vi "SelRess.vi"(5 "Instr":bool=TRUE, 6 "UsedRess":string[](array[string]), 7 "RessName":string caption="RessourceName", 8 "ErrorIn(No Error)":errorcluster caption="entrée d'erreur (pas d'erreur)", 9 "InstrNames":string[](array[string]), 10 "RessArray":string[][](array[string]), 11 "InstrName":string caption="Instrument Name") -> (0 "sortie d'erreur":errorcluster, 1 "RessAlias":string, 2 "RessNameOut":string, 3 "InstrNameOut":string, 4 "Cancel Out":bool)   [LabVIEW 2019]
uses:
  SelRessState.ctl
  <vilib>/Utility/miscctls.llb/LVRectTypeDef.ctl
panel:
  out "InstStep":string
  in  "Cancel":bool
  in  "Add":bool
  in  "Ressources":i32(listbox)
  # "1. Choose a ressource from the list to communicate with the Instrument\nor enter a ressource name manually"
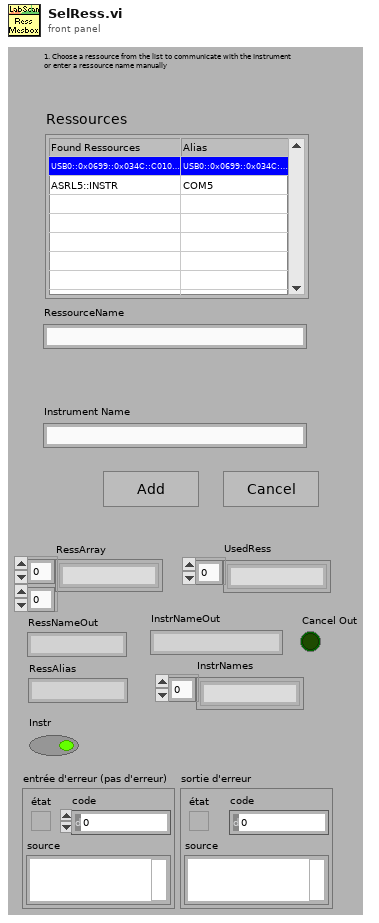
[diagram p1: front panel]
types:
  T1 = typedef "SelRessState.ctl" = enum16{"InitProg", "InstrNameExist?", "RessNameExist?", "RessInUse?", "RessSelected", "Cancel"}
  T2 = enum8{"Enabled", "Disabled", "Disabled and Grayed Out"}
  T3 = typedef "LVRectTypeDef.ctl" = cluster{"Left":i16, "Top":i16, "Right":i16, "Bottom":i16}
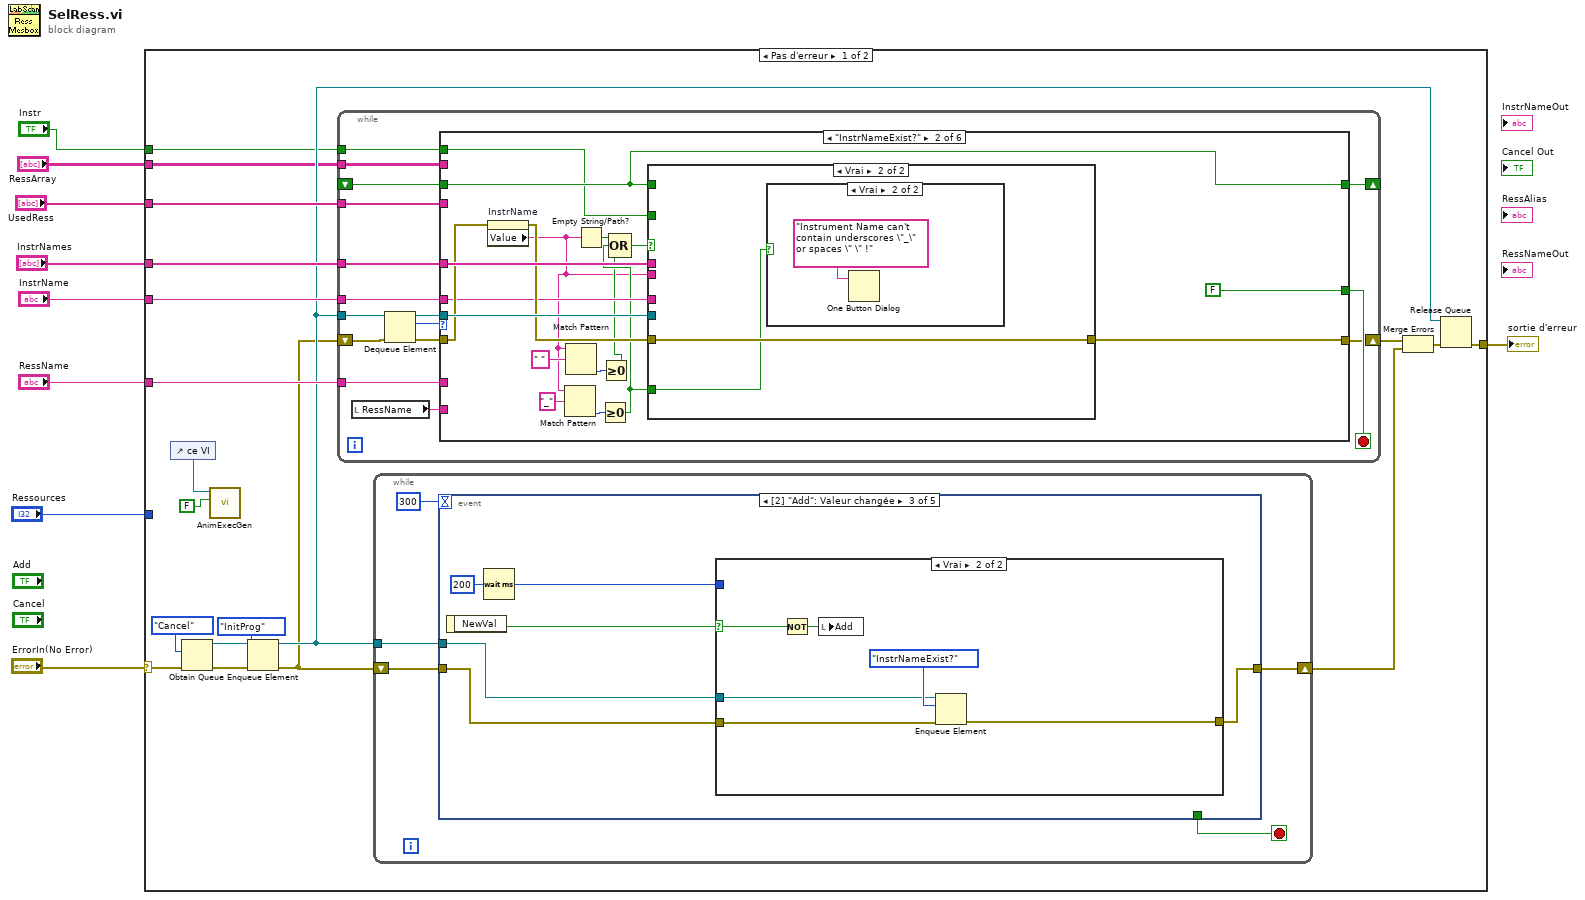
[diagram p0: block diagram]
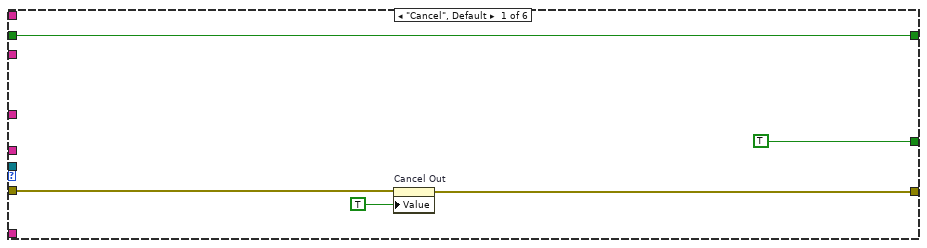
[diagram p2: hidden frame]
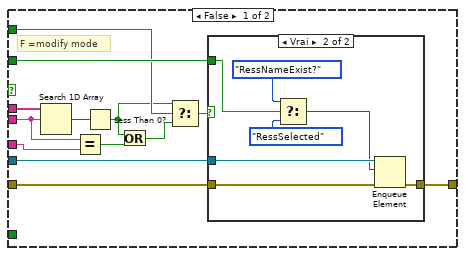
[diagram p3: hidden frame]
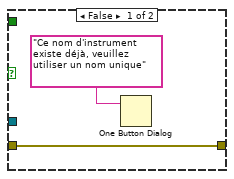
[diagram p4: hidden frame]
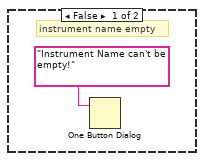
[diagram p5: hidden frame]
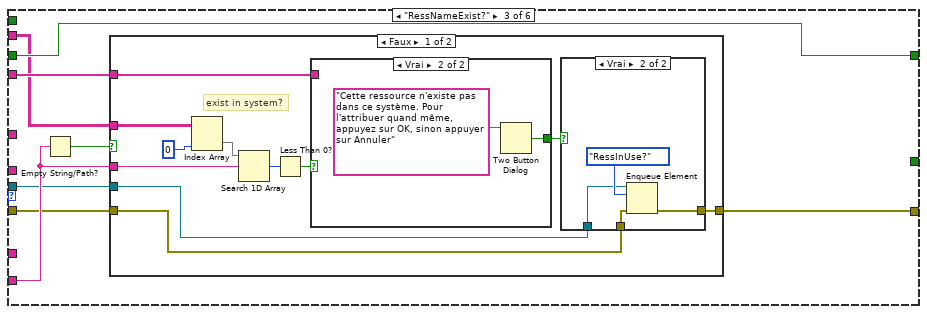
[diagram p6: hidden frame]
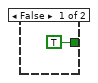
[diagram p8: hidden frame]
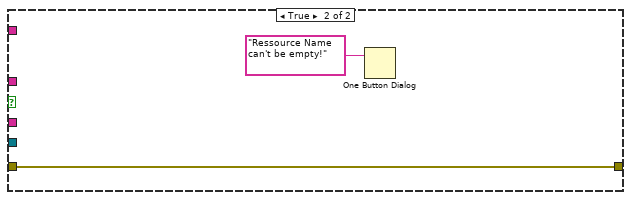
[diagram p9: hidden frame]
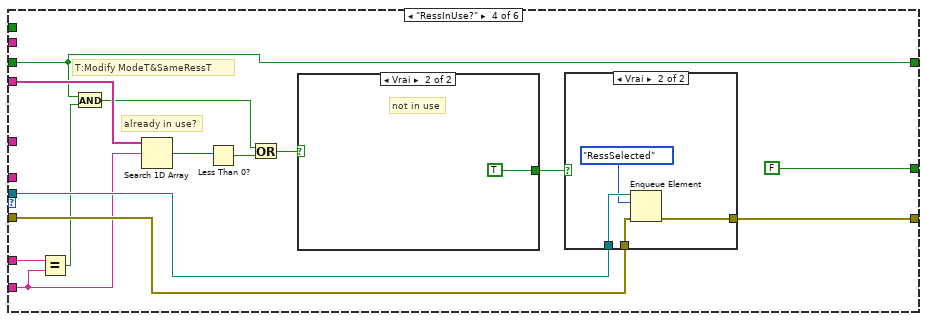
[diagram p10: hidden frame]
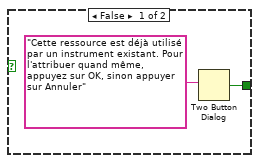
[diagram p12: hidden frame]
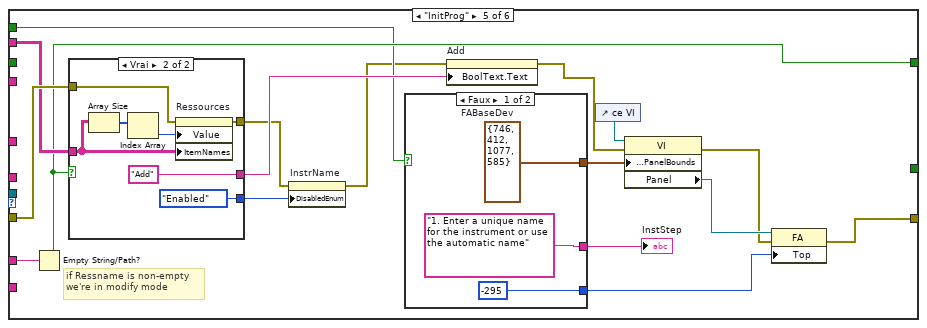
[diagram p13: hidden frame]
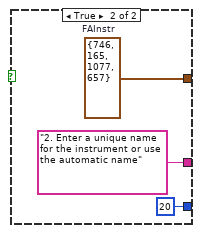
[diagram p14: hidden frame]
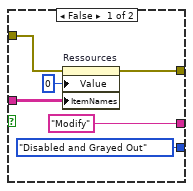
[diagram p15: hidden frame]
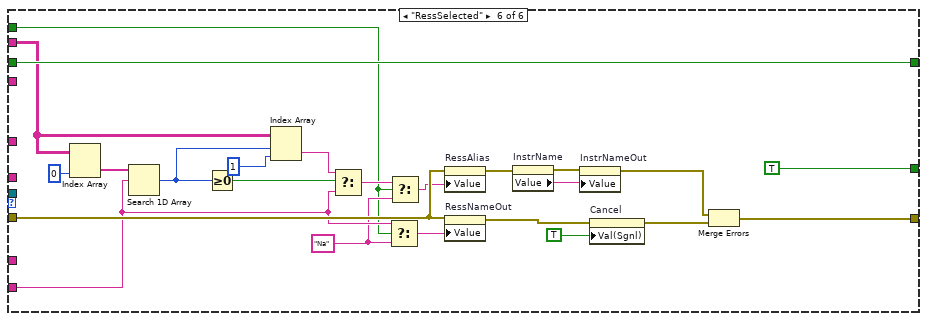
[diagram p16: hidden frame]
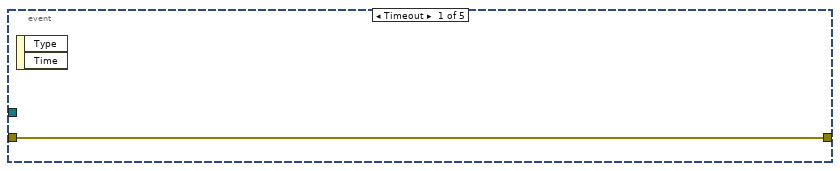
[diagram p17: hidden frame]
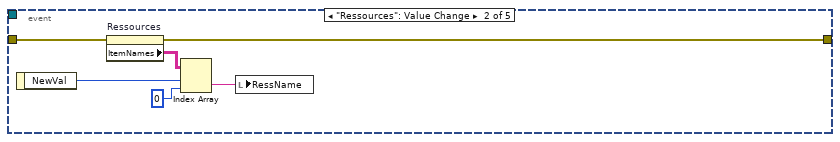
[diagram p18: hidden frame]
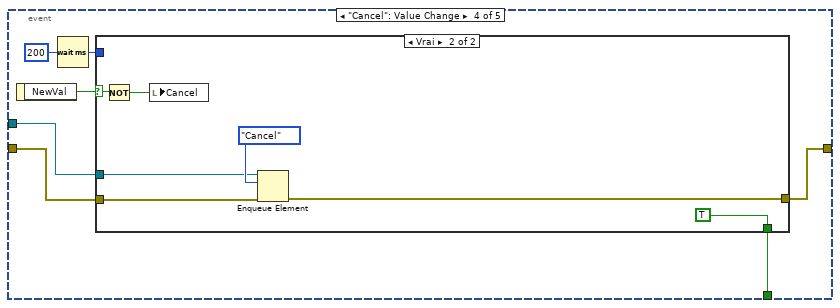
[diagram p20: hidden frame]
diagram:
  n1 = case shown="Pas d'erreur" "ErrorIn(No Error)" {
    selector: "ErrorIn(No Error)" -> [w28 w250]
    tunnel: [w21 w250] -> w8
    tunnel: "Ressources" -> [_ _]
    tunnel: "InstrNames" -> [w27 _]
    tunnel: "UsedRess" -> [w25 _]
    tunnel: "RessArray" -> [w13 _]
    tunnel: "InstrName" -> [w20 _]
    tunnel: "RessName" -> [w19 _]
    tunnel: "Instr" -> [w12 _]
    frame No Error {
      n2 = control-ref of="ce VI"() -> (w11:refnum<vi>)
      n3 = Obtain Queue(element data type=SelRessState."Cancel" ("Énum"), error in (no error)=w28) -> (queue out=w17:refnum<queue>, error out=w15:errorcluster)  [unwired: 3 in, 1 out]
      n4 = call <userlib>:"AnimExecGen.vi"("Animer l'exécution ?"=FALSE, "ViRef"=w11) -> ()  [unwired: 9 in, 1 out]
      n5 = Enqueue Element(queue=w17, element=SelRessState."InitProg" ("Énum"), error in (no error)=w15) -> (queue out=w18:refnum<queue>, error out=w14:errorcluster)  [unwired: 1 in, 1 out]
      n6 = while {
        tunnel: w18 -> [w43]
        tunnel: w27 -> [w42]
        tunnel: w25 -> [w39]
        shift-right: [w37] -> w24
        shift-left: w14 -> [w36]
        tunnel: w20 -> [w34]
        tunnel: w19 -> [w32]
        tunnel: w13 -> [w31]
        shift-right: [w30] -> _
        shift-left: _ -> [w35]
        tunnel: w12 -> [w29]
        stop <- w40 stop-if-true
        n7 = local read "RessName"() -> (w33:string)
        n8 = Dequeue Element(queue=w43, error in (no error)=w36) -> (queue out=w41:refnum<queue>, element=w44:T1, error out=w38:errorcluster)  [unwired: 1 in, 1 out]
        n9 = case shown="\"InstrNameExist?\"" w44 {
          tunnel: w42 -> [_ w67 _ _ _ _]
          tunnel: w41 -> [_ w65 w98 w131 _ _]
          tunnel: w33 -> [_ _ w100 w127 _ w185]
          tunnel: [TRUE ("T button?") FALSE ("T button?") _ FALSE ("T button?") _ TRUE ("T button?")] -> w40
          tunnel: w39 -> [_ _ w99 w136 _ _]
          tunnel: w38 -> [w47 w62 w96 w130 w160 w198]
          tunnel: [w46 w63 w97 w129 w148 w197] -> w37
          tunnel: w35 -> [w45 w59 w95 w123 _ w188]
          tunnel: w34 -> [_ w60 _ _ _ _]
          tunnel: w32 -> [_ _ _ w128 w161 _]
          tunnel: w31 -> [_ _ w94 _ w159 w187]
          tunnel: [w45 w59 w95 w123 w157 w188] -> w30
          tunnel: w29 -> [_ w58 _ _ w153 w181]
          frame "Cancel", Default {
            n10 = property on="Cancel Out" class="Bool (strict)"(error in=w47, "Value"=TRUE ("Cancel Out")) -> (error out=w46:errorcluster)  [unwired: 1 in, 1 out]
          }
          frame "InstrNameExist?" {
            n11 = property on="InstrName" class="Ch"(error in=w62) -> (error out=w61:errorcluster, "Value"=w50:string)  [unwired: 1 in, 1 out]
            n12 = Match Pattern(string=w50, regular expression="_" ("expression régulière")) -> (offset past match=w55:i32)  [unwired: 1 in, 3 out]
            n13 = Match Pattern(string=w50, regular expression=" " ("expression régulière")) -> (offset past match=w53:i32)  [unwired: 1 in, 3 out]
            n14 = Empty String/Path?(string/path=w50) -> (empty?=w66:bool)
            n15 = Greater Or Equal To 0?(x=w55) -> (x >= 0?=w54:bool)
            n16 = Greater Or Equal To 0?(x=w53) -> (x >= 0?=w51:bool)
            n17 = Compound Arithmetic op=OR ("Opérateur arithmétique")(w66, w54, w51) -> (w56:bool)
            n18 = case shown="Vrai" w56 {
              tunnel: w50 -> [w68 _]
              tunnel: w67 -> [w79 _]
              tunnel: w65 -> [w78 _]
              tunnel: [w77 w91] -> w63
              tunnel: w61 -> [w76 w91]
              tunnel: w59 -> [w71 _]
              tunnel: w60 -> [w74 _]
              tunnel: w58 -> [w72 _]
              tunnel: w54 -> [_ w90]
              frame False {
                # "F =modify mode"
                n19 = Search 1D Array(1D array=w79, element=w68) -> (index of element=w80:i32)  [unwired: 1 in]
                n20 = Equal?(x=w68, y=w74) -> (x = y?=w73:bool)
                n21 = Less Than 0?(x=w80) -> (x < 0?=w70:bool)
                n22 = Or(x=w70, y=w73) -> (x .or. y?=w69:bool)
                n23 = Select(t=w70, s=w71, f=w69) -> (s? t:f=w75:bool)
                n24 = case shown="Vrai" w75 {
                  tunnel: w78 -> [_ w89]
                  tunnel: [w81 w88] -> w77
                  tunnel: w76 -> [w81 w87]
                  tunnel: w72 -> [_ w86]
                  frame False {
                    n25 = One Button Dialog(message="Ce nom d'instrument existe déjà, veuillez utiliser un nom unique") -> ()  [unwired: 1 in, 1 out]
                  }
                  frame True {
                    n26 = Select(t=SelRessState."RessNameExist?" ("Énum"), s=w86, f=SelRessState."RessSelected" ("Énum")) -> (s? t:f=w83:T1)
                    n27 = Enqueue Element(queue=w89, element=w83, error in (no error)=w87) -> (error out=w88:errorcluster)  [unwired: 1 in, 2 out]
                  }
                }
              }
              frame True {
                n28 = case shown="Vrai" w90 {
                  frame False {
                    # "instrument name empty"
                    n29 = One Button Dialog(message="Instrument Name can't be empty!") -> ()  [unwired: 1 in, 1 out]
                  }
                  frame True {
                    n30 = One Button Dialog(message="Instrument Name can't contain underscores \"_\" or spaces \" \" !") -> ()  [unwired: 1 in, 1 out]
                  }
                }
              }
            }
          }
          frame "RessNameExist?" {
            n31 = Empty String/Path?(string/path=w100) -> (empty?=w101:bool)
            n32 = case shown="Faux" w101 {
              tunnel: w100 -> [w108 _]
              tunnel: w99 -> [w107 _]
              tunnel: w98 -> [w103 _]
              tunnel: [w104 w121] -> w97
              tunnel: w96 -> [w102 w121]
              tunnel: w94 -> [w106 _]
              frame False {
                # "exist in system?"
                n33 = Index Array(array=w106, index (col)=0 ("indice désactivé (col)")) -> (element=w111:string[])  [unwired: 1 in]
                n34 = Search 1D Array(1D array=w111, element=w108) -> (index of element=w110:i32)  [unwired: 1 in]
                n35 = Less Than 0?(x=w110) -> (x < 0?=w109:bool)
                n36 = case shown="Vrai" w109 {
                  tunnel: w107 -> [_ _]
                  tunnel: [TRUE ("T button?") w119] -> w105
                  frame False {
                  }
                  frame True {
                    n37 = Two Button Dialog(message="Cette ressource n'existe pas dans ce système. Pour l'attribuer quand même, appuyez sur OK, sinon appuyer sur Annuler") -> (T button?=w119:bool)  [unwired: 2 in]
                  }
                }
                n38 = case shown="Vrai" w105 {
                  tunnel: [w113 w116] -> w104
                  tunnel: w103 -> [_ w115]
                  tunnel: w102 -> [w113 w114]
                  frame False {
                  }
                  frame True {
                    n39 = Enqueue Element(queue=w115, element=SelRessState."RessInUse?" ("Énum"), error in (no error)=w114) -> (error out=w116:errorcluster)  [unwired: 1 in, 2 out]
                  }
                }
              }
              frame True {
                n40 = One Button Dialog(message="Ressource Name can't be empty!") -> ()  [unwired: 1 in, 1 out]
              }
            }
          }
          frame "RessInUse?" {
            # "T:Modify ModeT&SameRessT"
            # "already in use?"
            n41 = Equal?(x=w128, y=w127) -> (x = y?=w126:bool)
            n42 = And(x=w123, y=w126) -> (x .and. y?=w124:bool)
            n43 = Search 1D Array(1D array=w136, element=w127) -> (index of element=w135:i32)  [unwired: 1 in]
            n44 = Less Than 0?(x=w135) -> (x < 0?=w134:bool)
            n45 = Or(x=w124, y=w134) -> (x .or. y?=w125:bool)
            n46 = case shown="Vrai" w125 {
              tunnel: [w142 TRUE] -> w132
              frame False {
                n47 = Two Button Dialog(message="Cette ressource est déjà utilisé par un instrument existant. Pour l'attribuer quand même, appuyez sur OK, sinon appuyer sur Annuler") -> (T button?=w142:bool)  [unwired: 2 in]
              }
              frame True {
                # "not in use"
              }
            }
            n48 = case shown="Vrai" w132 {
              tunnel: w131 -> [_ w141]
              tunnel: w130 -> [w137 w139]
              tunnel: [w137 w138] -> w129
              frame False {
              }
              frame True {
                n49 = Enqueue Element(queue=w141, element=SelRessState."RessSelected" ("Énum"), error in (no error)=w139) -> (error out=w138:errorcluster)  [unwired: 1 in, 2 out]
              }
            }
          }
          frame "InitProg" {
            # "if Ressname is non-empty\nwe're in modify mode"
            n50 = Empty String/Path?(string/path=w161) -> (empty?=w157:bool)
            n51 = case shown="Vrai" w157 {
              tunnel: [w172 w180] -> w147
              tunnel: w160 -> [w171 w179]
              tunnel: w159 -> [w169 w176]
              tunnel: ["Modify" "Add"] -> w158
              tunnel: [T2."Disabled and Grayed Out" ("Désactivé") T2."Enabled" ("Désactivé")] -> w145
              frame False {
                n52 = property on="Ressources" class="ListeMCol (strict)"(error in=w171, "Value"=0 ("Valeur (Signalisation)"), "ItemNames"=w169) -> (error out=w172:errorcluster)  [unwired: 1 in, 1 out]
              }
              frame True {
                n53 = Array Size(array=w176) -> (size(s)=w175:i32[])
                n54 = Index Array(array=w175) -> (element=w174:i32)  [unwired: 1 in]
                n55 = property on="Ressources" class="ListeMCol (strict)"(error in=w179, "Value"=w174, "ItemNames"=w176) -> (error out=w180:errorcluster)  [unwired: 1 in, 1 out]
              }
            }
            n56 = property on="InstrName" class="Ch"(error in=w147, "DisabledEnum"=w145) -> (error out=w146:errorcluster)  [unwired: 1 in, 1 out]
            n57 = case shown="Faux" w153 {
              tunnel: ["1. Enter a unique name for the instrument or use the automatic name" ("InstStep") "2. Enter a unique name for the instrument or use the automatic name" ("InstStep")] -> w154
              tunnel: [w163 w166] -> w152
              tunnel: [-295 ("Position : haut") 20 ("Position : haut")] -> w150
              frame False {
                w163 = T3 {"Left"=746, "Top"=412, "Right"=1077, "Bottom"=585}  # FABaseDev
              }
              frame True {
                w166 = T3 {"Left"=746, "Top"=165, "Right"=1077, "Bottom"=657}  # FAInstr
              }
            }
            "InstStep" <- w154
            n58 = property on="Add" class="Bool (strict)"(error in=w146, "BoolText.Text"=w158) -> (error out=w155:errorcluster)  [unwired: 1 in, 1 out]
            n59 = control-ref of="ce VI"() -> (w156:refnum<vi>)
            n60 = property class="VI"(reference=w156, error in=w155, "Front Panel.PanelBounds"=w152) -> (error out=w149:errorcluster, "Panel"=w151:refnum<vi>)  [unwired: 1 out]
            n61 = property class="FA"(reference=w151, error in=w149, "Top"=w150) -> (error out=w148:errorcluster)  [unwired: 1 out]
          }
          frame "RessSelected" {
            w184 = "Na" ("cas faux")
            n62 = Index Array(array=w187, index (col)=0 ("indice désactivé (col)")) -> (element=w202:string[])  [unwired: 1 in]
            n63 = Search 1D Array(1D array=w202, element=w185) -> (index of element=w201:i32)  [unwired: 1 in]
            n64 = Greater Or Equal To 0?(x=w201) -> (x >= 0?=w200:bool)
            n65 = Index Array(array=w187, index (row)=w201, index (col)=1 ("indice désactivé (col)")) -> (element=w199:string)
            n66 = Select(t=w199, s=w200, f=w185) -> (s? t:f=w186:string)
            n67 = Select(t=w185, s=w181, f=w184) -> (s? t:f=w182:string)
            n68 = Select(t=w186, s=w181, f=w184) -> (s? t:f=w183:string)
            n69 = property on="RessAlias" class="Ch"(error in=w198, "Value"=w183) -> (error out=w191:errorcluster)  [unwired: 1 in, 1 out]
            n70 = property on="RessNameOut" class="Ch"(error in=w198, "Value"=w182) -> (error out=w195:errorcluster)  [unwired: 1 in, 1 out]
            n71 = property on="InstrName" class="Ch"(error in=w191) -> (error out=w190:errorcluster, "Value"=w189:string)  [unwired: 1 in, 1 out]
            n72 = property on="InstrNameOut" class="Ch"(error in=w190, "Value"=w189) -> (error out=w192:errorcluster)  [unwired: 1 in, 1 out]
            n73 = property on="Cancel" class="Bool (strict)"(error in=w195, "Val(Sgnl)"=TRUE ("Valeur (Signalisation)")) -> (error out=w194:errorcluster)  [unwired: 1 in, 1 out]
            n74 = Merge Errors(w192, w194) -> (w197:errorcluster)
          }
        }
      }
      n75 = while {
        shift-right: [w208] -> w23
        shift-left: w14 -> [w207]
        tunnel: w18 -> [w206]
        stop <- w205 stop-if-true
        n76 = event shown="[2] \"Add\": Valeur changée" {
          selector: _ -> [_ _ _ _ _]
          dyn-events: _ -> [_ _ _ _ _]
          timeout: 300 ("attente (ms)") -> [_ _ _ _ _]
          tunnel: [w210 w211 w217 w232 w247] -> w208
          tunnel: w207 -> [w210 w212 w218 w233 w248]
          tunnel: w206 -> [_ _ w219 w230 w249]
          tunnel: [_ _ _ w231 TRUE ("x")] -> w205
          event Timeout {
            n77 = event-data() -> ()  [unwired: 1 in, 2 out]
          }
          event "Ressources": Value Change {
            n78 = event-data() -> ("NewVal"=w213:i32)  [unwired: 1 in]
            n79 = property on="Ressources" class="ListeMCol (strict)"(error in=w212) -> (error out=w211:errorcluster, "ItemNames"=w216:string[][])  [unwired: 1 in, 1 out]
            n80 = Index Array(array=w216, index (row)=w213, index (col)=0 ("indice désactivé (col)")) -> (element=w214:string)
            n81 = local write "RessName"(w214) -> ()
          }
          event "Add": Value Change {
            n82 = event-data() -> ("NewVal"=w222:bool)  [unwired: 1 in]
            n83 = Wait (ms)(milliseconds to wait=u32 200 ("attente (ms)")) -> (millisecond timer value=w221:u32)
            n84 = case shown="Vrai" w222 {
              selector: w222 -> [_ w229]
              tunnel: w221 -> [_ _]
              tunnel: w219 -> [_ w226]
              tunnel: w218 -> [w223 w225]
              tunnel: [w223 w224] -> w217
              frame False {
              }
              frame True {
                n85 = Not(x=w229) -> (.not. x?=w228:bool)
                n86 = local write "Add"(w228) -> ()
                n87 = Enqueue Element(queue=w226, element=SelRessState."InstrNameExist?" ("Énum"), error in (no error)=w225) -> (error out=w224:errorcluster)  [unwired: 1 in, 2 out]
              }
            }
          }
          event "Cancel": Value Change {
            n88 = event-data() -> ("NewVal"=w236:bool)  [unwired: 1 in]
            n89 = Wait (ms)(milliseconds to wait=u32 200 ("attente (ms)")) -> (millisecond timer value=w235:u32)
            n90 = case shown="Vrai" w236 {
              selector: w236 -> [_ w244]
              tunnel: w235 -> [_ _]
              tunnel: w230 -> [_ w241]
              tunnel: w233 -> [w237 w240]
              tunnel: [w237 w239] -> w232
              tunnel: [_ TRUE ("x")] -> w231
              frame False {
              }
              frame True {
                n91 = Not(x=w244) -> (.not. x?=w243:bool)
                n92 = local write "Cancel"(w243) -> ()
                n93 = Enqueue Element(queue=w241, element=SelRessState."Cancel" ("Énum"), error in (no error)=w240) -> (error out=w239:errorcluster)  [unwired: 1 in, 2 out]
              }
            }
          }
          event Panel Close {
            n94 = event-data() -> ()  [unwired: 1 in, 1 out]
            n95 = Enqueue Element(queue=w249, element=SelRessState."Cancel" ("Énum"), error in (no error)=w248) -> (error out=w247:errorcluster)  [unwired: 1 in, 2 out]
          }
        }
      }
      n96 = Merge Errors(w24, w23) -> (w22:errorcluster)
      n97 = Release Queue(queue=w18, error in (no error)=w22) -> (error out=w21:errorcluster)  [unwired: 1 in, 2 out]
    }
    frame Error {
    }
  }
  "sortie d'erreur" <- w8
